vi "String Hex to String Binary.vi"() -> ()   [LabVIEW 2015]
panel:
  out "Number (Binary format)":u64 format="%064b"
  out "Binary String":string
  in  "Hexadecimal String":string="8300000000008002"
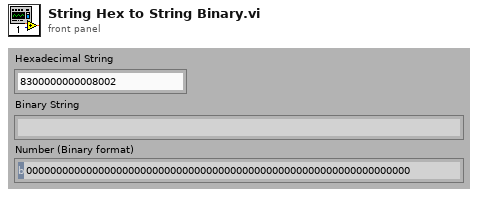
[diagram p1: front panel]
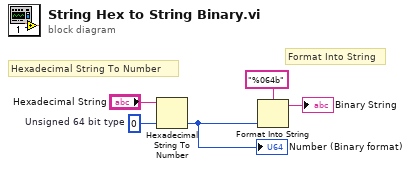
[diagram p0: block diagram]
diagram:
  w1 = u64 0  # Unsigned 64 bit type
  # "Format Into String"
  # "Hexadecimal String To Number"
  n1 = Hexadecimal String To Number(string="Hexadecimal String", default (0uL)=w1) -> (number=w4:u64)  [unwired: 1 in, 1 out]
  "Number (Binary format)" <- w4
  n2 = Format Into String(format string="%064b", w4) -> (resulting string=→"Binary String":string)  [unwired: 2 in, 1 out]
